vi "controllerMain.vi"(8 "error in (no error)":errorcluster, 10 "UserEvents in":refnum<class "UserEvents.lvclass">, 11 "Controller in":refnum<class "Controller.lvclass">) -> (0 "error out":errorcluster, 3 "Controller out":refnum<class "Controller.lvclass">)   [LabVIEW 2013, in "Controller.lvclass"]
uses:
  Controller.lvclass
  UserEvents/UserEvents.lvclass
  StateFactory/StateFactory.lvclass
  Typedefs/StateSelector.ctl
  Model/Model/Model.lvclass
  Context/Context.lvclass
  CommandFactory/CommandFactory.lvclass
  Model/SDAFactory/SDAFactory.lvclass
  <userlib>/Common/SerialProtocols/SerialCommFactory/SerialCommFactory/SerialCommFactory.lvclass
  <vilib>/Platform/TimedLoop/XDataNode/timing_clust.ctl
  <vilib>/Platform/TimedLoop/XDataNode/nitl_modes.ctl
  <vilib>/Platform/TimedLoop/XDataNode/wakeup.ctl
  UserEvents/UserEvents.lvclass/UserEvents.ctl
  Model/Model/Model.lvclass/Model.ctl
  Context/Context.lvclass/Context.ctl
  Typedefs/CommandSelector.ctl
  Command/Command.lvclass
  <vilib>/platform/TimedLoop/XDataNode/XDataNode.xnode
  <vilib>/Platform/TimedLoop/XDataNode/XDNodeRunTimeDep.lvlib
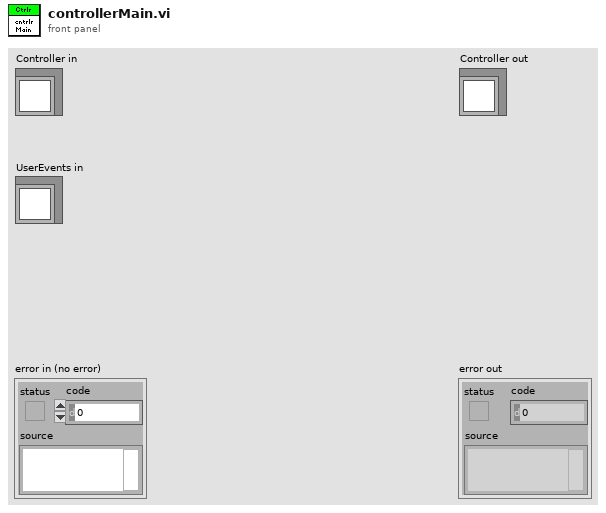
[diagram p1: front panel]
types:
  T1 = typedef "StateSelector.ctl" = enum16{"DataOnDemandState", "DataStreamingState", "FaultState", "OffState", "StandbyState"}
  T2 = typedef "PubDataEvents.ctl" = cluster{"State":refnum<user-event>, "ErrorCode":refnum<user-event>, "OutputData":refnum<user-event>, "InputData":refnum<user-event>, "ILCConfig":refnum<user-event>, "NeedUserOutputs":refnum<user-event>}
  T3 = typedef "SubDataEvents.ctl" = cluster{"Command":refnum<user-event>}
  T4 = typedef "XDNodeRunTimeDep.lvlib/timing_clust.ctl" = cluster{"Expected End [f-1]":u64, "Actual End [f-1]":u64, "Finished Late? [f-1]":bool, "Expected End [i-1]":u64, "Actual End [i-1]":u64, "Finished Late? [i-1]":bool, "Expected Start [i]":u64, "Actual Start [i]":u64, "Expected Start [f]":u64, "Actual Start [f]":u64, "Source Name":string, "Structure Name":string, "Period":i64, "Deadline":i64, "Offset":i64, "Start":i64, "Priority":i32, "Timeout":i32, "Mode":T5, "Wakeup Reason":T6, "Error":errorcluster, "Source Type":string, "Secondary Source Type":string, "Global End Time":u64, "Global Start Time":u64, "Frame Duration":u64, "Iteration Duration":u64, "Assigned CPU":i32, "I/O Scan Engine Mode":u32}
  T5 = typedef "XDNodeRunTimeDep.lvlib/nitl_modes.ctl" = enum32{"No Change", "Process missed periods, maintain original phase", "Discard missed periods, maintain original phase", "Process missed periods, ignore original phase", "Discard missed periods, ignore original phase"}
  T6 = typedef "XDNodeRunTimeDep.lvlib/wakeup.ctl" = enum32{"Normal", "Aborted", "Asynchronous wakeup", "Timing source error", "Timed loop error", "Timeout"}
  T7 = typedef "CommandSelector.ctl" = enum16{"ClearError", "Exit", "StandBy", "Start", "SwitchToOnDemandMode", "SwitchToStreamMode", "Update"}
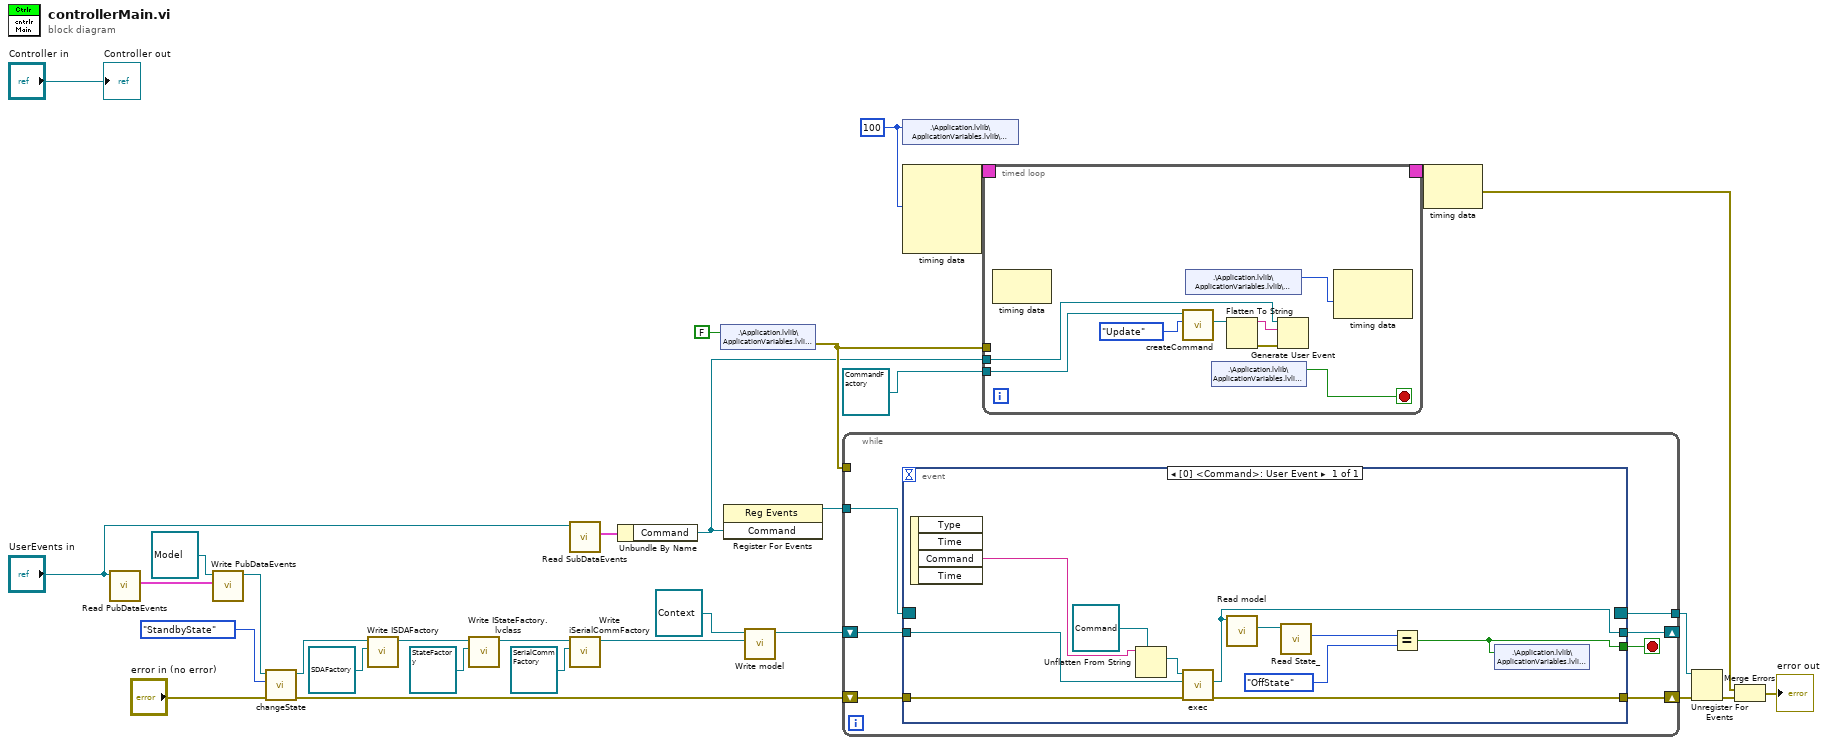
[diagram p0: block diagram]
diagram:
  w4 = i64 100 ("Period")
  n1 = call "Read PubDataEvents.vi"("UserEvents in"="UserEvents in") -> ("PubDataEvents"=w9:T2)  [unwired: 9 in, 1 out]
  n2 = call "Write PubDataEvents.vi"("PubDataEvents"=w9, "Model in"=refnum<class "Model.lvclass"> refnum) -> ("Model out"=w12:refnum<class "Model.lvclass">)  [unwired: 9 in]
  n3 = call "changeState.vi"("error in (no error)"="error in (no error)", "State:"=StateSelector."StandbyState", "Model in"=w12) -> ("error out"=w14:errorcluster, "Model out"=w21:refnum<class "Model.lvclass">)  [unwired: 7 in]
  n4 = call "Write ISDAFactory.vi"("ISDAFactory.lvclass"=refnum<class "SDAFactory.lvclass"> refnum ("SDAFactory.lvclass"), "Model in"=w21) -> ("Model out"=w20:refnum<class "Model.lvclass">)  [unwired: 9 in]
  n5 = call "Write IStateFactory.lvclass.vi"("IStateFactory.lvclass"=refnum<class "StateFactory.lvclass"> refnum ("StateFactory.lvclass"), "Model in"=w20) -> ("Model out"=w3:refnum<class "Model.lvclass">)  [unwired: 9 in]
  n6 = call "Read SubDataEvents.vi"("UserEvents in"="UserEvents in") -> ("SubDataEvents"=w18:T3)  [unwired: 9 in, 1 out]
  n7 = call "Write iSerialCommFactory.vi"("ISerialCommFactory.lvclass"=refnum<class "SerialCommFactory.lvclass"> refnum ("SerialCommFactory.lvclass"), "Model in"=w3) -> ("Model out"=w2:refnum<class "Model.lvclass">)  [unwired: 9 in]
  n8 = Unbundle By Name(w18) -> ("Command"=w6:refnum<user-event>)
  n9 = shared-variable ".\\Application.lvlib\\ApplicationVariables.lvlib\\ExitIsTrue"(FALSE ("ExitIsTrue")) -> (error out=w22:errorcluster)  [unwired: 1 in]
  n10 = register-events(w6) -> (reference out=w17:refnum<event-registration>)  [unwired: 2 in, 1 out]
  n11 = call "Write model.vi"("Model.lvclass"=w2, "Context in"=refnum<class "Context.lvclass"> refnum ("Context.lvclass")) -> ("Context out"=w28:refnum<class "Context.lvclass">)  [unwired: 9 in]
  n12 = while {
    shift-right: [w37] -> w15
    shift-left: w14 -> [w34]
    shift-right: [w36] -> _
    shift-left: w28 -> [w38]
    tunnel: w22 -> [_]
    tunnel: w17 -> [w33]
    tunnel: [w32] -> w16
    stop <- w35 stop-if-true
    n13 = event shown="[0] <Command>: User Event" {
      selector: w33 -> [_]
      dyn-events: [_] -> w32
      timeout: _ -> [_]
      tunnel: w38 -> [w47]
      tunnel: [w44] -> w37
      tunnel: [w43] -> w36
      tunnel: [w42] -> w35
      tunnel: w34 -> [w40]
      event User Event {
        n14 = event-data() -> ("Command"=w39:string)  [unwired: 1 in, 3 out]
        n15 = Unflatten From String(type=refnum<class "Command.lvclass"> refnum ("Command.lvclass"), binary string=w39) -> (value=w48:refnum<class "Command.lvclass">)  [unwired: 3 in, 2 out]
        n16 = call-dynamic "exec.vi"("error in (no error)"=w40, "context"=w47, "Command in"=w48) -> ("error out"=w44:errorcluster, "context 2"=w43:refnum<class "Context.lvclass">)  [unwired: 6 in, 1 out]
        n17 = call "Read model.vi"("Context in"=w43) -> ("Model.lvclass"=w46:refnum<class "Model.lvclass">)  [unwired: 9 in, 1 out]
        n18 = call "Read State_.vi"("Model in"=w46) -> ("State:"=w41:T1)  [unwired: 9 in, 1 out]
        n19 = Equal?(x=w41, y=StateSelector."OffState") -> (x = y?=w42:bool)
        n20 = shared-variable ".\\Application.lvlib\\ApplicationVariables.lvlib\\ExitIsTrue"(w42) -> ()  [unwired: 1 in, 1 out]
      }
    }
  }
  n21 = shared-variable ".\\Application.lvlib\\ApplicationVariables.lvlib\\LoopRate_ms"(w4) -> ()  [unwired: 1 in, 1 out]
  n22 = node-c288(w4) -> (w24:T4)  [unwired: 3 in]
  n23 = timed-loop {
    timing: w24 -> [_]
    timing-out: [_] -> w23
    tunnel: refnum<class "CommandFactory.lvclass"> refnum ("CommandFactory.lvclass") -> [w56]
    tunnel: w22 -> [_]
    tunnel: w6 -> [w52]
    stop <- w54 stop-if-true
    n24 = node-c288() -> ()  [unwired: 1 in, 1 out]
    n25 = call-dynamic "createCommand.vi"("Command"=CommandSelector."Update", "CommandFactory in"=w56) -> ("command"=w55:refnum<class "Command.lvclass">)  [unwired: 7 in, 2 out]
    n26 = shared-variable ".\\Application.lvlib\\ApplicationVariables.lvlib\\LoopRate_ms"() -> (w50:i64)  [unwired: 1 in, 1 out]
    n27 = shared-variable ".\\Application.lvlib\\ApplicationVariables.lvlib\\ExitIsTrue"() -> (w54:bool)  [unwired: 1 in, 1 out]
    n28 = Flatten To String(anything=w55) -> (data string=w51:string, error out=w53:errorcluster)  [unwired: 3 in, 1 out]
    n29 = Generate User Event(user event=w52, event data cluster=w51, error in=w53) -> ()  [unwired: 1 in, 2 out]
    n30 = node-c288(w50) -> ()  [unwired: 1 in, 1 out]
  }
  n31 = node-c288(w23) -> (w8:errorcluster)
  n32 = Unregister For Events(event registration refnum=w16, error in=w15) -> (error out=w7:errorcluster)
  n33 = Merge Errors(w8, w7) -> (→"error out":errorcluster)
  "Controller out" <- "Controller in"
